vi "LIA_FPGA.vi"() -> ()   [LabVIEW 2009]
uses:
  <vilib>/LabVIEW Targets/FPGA/cRIO/shared/nicrio_ModuleControls/nicrio_cRIO-9233_DataRatesRing.ctl
  <vilib>/rvi/LocalResourceManager/LocalResourceManager.xnode
  <vilib>/rvi/eio/common/nirviEmuReportErrorAndStop.vi
  <vilib>/rvi/DataTransferAndStorage/Container/Common/niFpgaContainerSetEmuInfo.vi
  <vilib>/rvi/DataTransferAndStorage/Container/Common/niFpgaContainerState.ctl
  <vilib>/rvi/DataTransferAndStorage/Container/Common/niFpgaDataTypeControl.ctl
  <vilib>/rvi/DataTransferAndStorage/Container/Common/niFpgaContainerImplementationControl.ctl
  <vilib>/rvi/DataTransferAndStorage/Container/Common/niFpgaContainerArbitrationOptionsControl.ctl
  <vilib>/rvi/DataTransferAndStorage/Container/Common/niFpgaTransferTypeControl.ctl
  <vilib>/rvi/DataTransferAndStorage/Container/Common/niFpgaContainerInitializationParameters.ctl
  <vilib>/rvi/DataTransferAndStorage/Container/Common/niFpgaContainerMetaDataKey.ctl
  <vilib>/eio/EIOPropertyNode/EIOPropertyNode.xnode
  <vilib>/rvi/eio/nirviEIOPropertyImplementation/nirviEIOPropertyImplementation.xnode
  <vilib>/rvi/eio/common/nirviEmuTemplatePropertyGet_noerrors.vi
  <vilib>/rvi/eio/common/nirviEmuTemplatePropertySet_noerrors.vi
  <vilib>/eio/EIONode/EIONode.xnode
  <vilib>/rvi/eio/nirviEIOImplementation/nirviEIOImplementation.xnode
  <vilib>/rvi/eio/common/nirviEmuTemplateMethod_noerrors.vi
  <vilib>/rvi/eio/common/nirviEmuClasses.ctl
  <vilib>/Platform/TimedLoop/XDataNode/XDataNode.xnode
  <vilib>/Platform/TimedLoop/XDataNode/loadlvalarms.vi
  <vilib>/Platform/TimedLoop/XDataNode/timing_clust.ctl
  <vilib>/Platform/TimedLoop/XDataNode/nitl_modes.ctl
  <vilib>/Platform/TimedLoop/XDataNode/wakeup.ctl
  <vilib>/rvi/DataTransferAndStorage/Container/XNode/niFpgaContainer.xnode
  <vilib>/rvi/FIFO/Fifo_Resource/nirvififoUniquifyingName.vi
  <vilib>/rvi/FXPMathLib/FxpSinAndCos/XNode/nifxpmath_SinAndCos.xnode
  <vilib>/rvi/FXPMathLib/FxpSinAndCos/subVIs/nifxpmath_SinAndCos_SimConfig.ctl
  <vilib>/rvi/FXPMathLib/FxpSinAndCos/simVIs/DllFxpSinAndCosTemp_sub.vi
  <vilib>/rvi/interface/RandomDataEmulation/niFpgaRandomDataHandleErrors.vi
  <vilib>/rvi/interface/RandomDataEmulation/nirviRandomDataFPGAFIFO.vi
  <vilib>/rvi/DataTransferAndStorage/Container/Common/niFpgaContainerMethod.ctl
  <vilib>/Platform/TimedLoop/XDataNode/XDNodeRunTimeDep.lvlib
panel:
  in  "dec":i32
  out "channelQ":i64
  out "channelI":i64
  in  "reset":bool
  in  "Data Rate":T1=2 items=["50.000 kS/s (NI 9233)"=2, "33.333 kS/s (NI 9233)"=3, "25.000 kS/s (NI 9233)"=34, "16.667 kS/s (NI 9233)"=35, "12.500 kS/s (NI 9233)"=36, "10.000 kS/s (NI 9233)"=37, "  8.333 kS/s (NI 9233)"=38, "  7.143 kS/s (NI 9233)"=39, "  6.250 kS/s (NI 9233)"=40, "  5.556 kS/s (NI 9233)"=41, "  5.000 kS/s (NI 9233)"=42, "  4.545 kS/s (NI 9233)"=43, "  4.167 kS/s (NI 9233)"=44, "  3.846 kS/s (NI 9233)"=45, "  3.571 kS/s (NI 9233)"=46, "  3.333 kS/s (NI 9233)"=47, "  3.125 kS/s (NI 9233)"=48, "  2.941 kS/s (NI 9233)"=49, "  2.778 kS/s (NI 9233)"=50, "  2.632 kS/s (NI 9233)"=51, "  2.500 kS/s (NI 9233)"=52, "  2.381 kS/s (NI 9233)"=53, "  2.273 kS/s (NI 9233)"=54, "  2.174 kS/s (NI 9233)"=55, "  2.083 kS/s (NI 9233)"=56, "  2.000 kS/s (NI 9233)"=57]
  out "f_2":fxp<+/-,32,0> format="%.32g"
  out "f":fxp<+/-,32,0> format="%.32g"
  out "Offset":i32
  out "LSB Weight":u32
  in  "channel":i16
  in  "test":bool
  out "error":bool
  in  "dec2":i16
  in  "K":fxp<+,16,0>
  in  "nominal freq":fxp<+,16,0>
  in  "dec1":i16
  in  "stages":i8=1
  in  "stop":bool
  in  "decimation":i16=1024
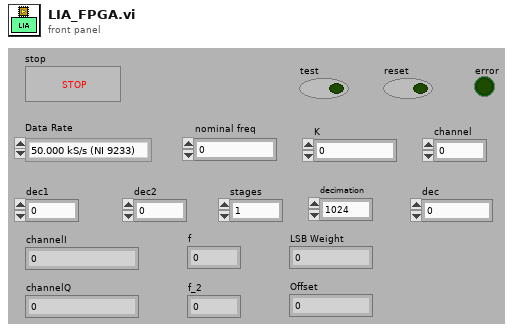
[diagram p1: front panel]
types:
  T1 = typedef "nicrio_cRIO-9233_DataRatesRing.ctl" = u8
  T2 = typedef "nirviEmuClasses.ctl" = enum16{"IO Read", "IO Write", "Method", "Property Read", "Property Write"}
  T3 = typedef "XDNodeRunTimeDep.lvlib/timing_clust.ctl" = cluster{"Expected End [f-1]":u64, "Actual End [f-1]":u64, "Finished Late? [f-1]":bool, "Expected End [i-1]":u64, "Actual End [i-1]":u64, "Finished Late? [i-1]":bool, "Expected Start [i]":u64, "Actual Start [i]":u64, "Expected Start [f]":u64, "Actual Start [f]":u64, "Source Name":string, "Structure Name":string, "Period":i64, "Deadline":i64, "Offset":i64, "Start":i64, "Priority":i32, "Timeout":i32, "Mode":T4, "Wakeup Reason":T5, "Error":errorcluster, "Source Type":string, "Secondary Source Type":string, "Global End Time":u64, "Global Start Time":u64, "Frame Duration":u64, "Iteration Duration":u64, "Assigned CPU":i32, "I/O Scan Engine Mode":u32}
  T4 = typedef "XDNodeRunTimeDep.lvlib/nitl_modes.ctl" = enum32{"No Change", "Process missed periods, maintain original phase", "Discard missed periods, maintain original phase", "Process missed periods, ignore original phase", "Discard missed periods, ignore original phase"}
  T5 = typedef "XDNodeRunTimeDep.lvlib/wakeup.ctl" = enum32{"Normal", "Aborted", "Asynchronous wakeup", "Timing source error", "Timed loop error", "Timeout"}
  T6 = typedef "niFpgaContainerMethod.ctl" = enum16{"Write", "Read", "Clear", "Get Number of Elements to Write", "Get Number of Elements to Read", "Enable", "Disable", "Flush and Disable", "Get Stream State"}
  T7 = typedef "niFpgaTransferTypeControl.ctl" = enum16{"Target-Scoped", "Host to Target - DMA", "Target to Host - DMA", "Peer to Peer Reader", "Peer to Peer Writer", "Bidirectional"}
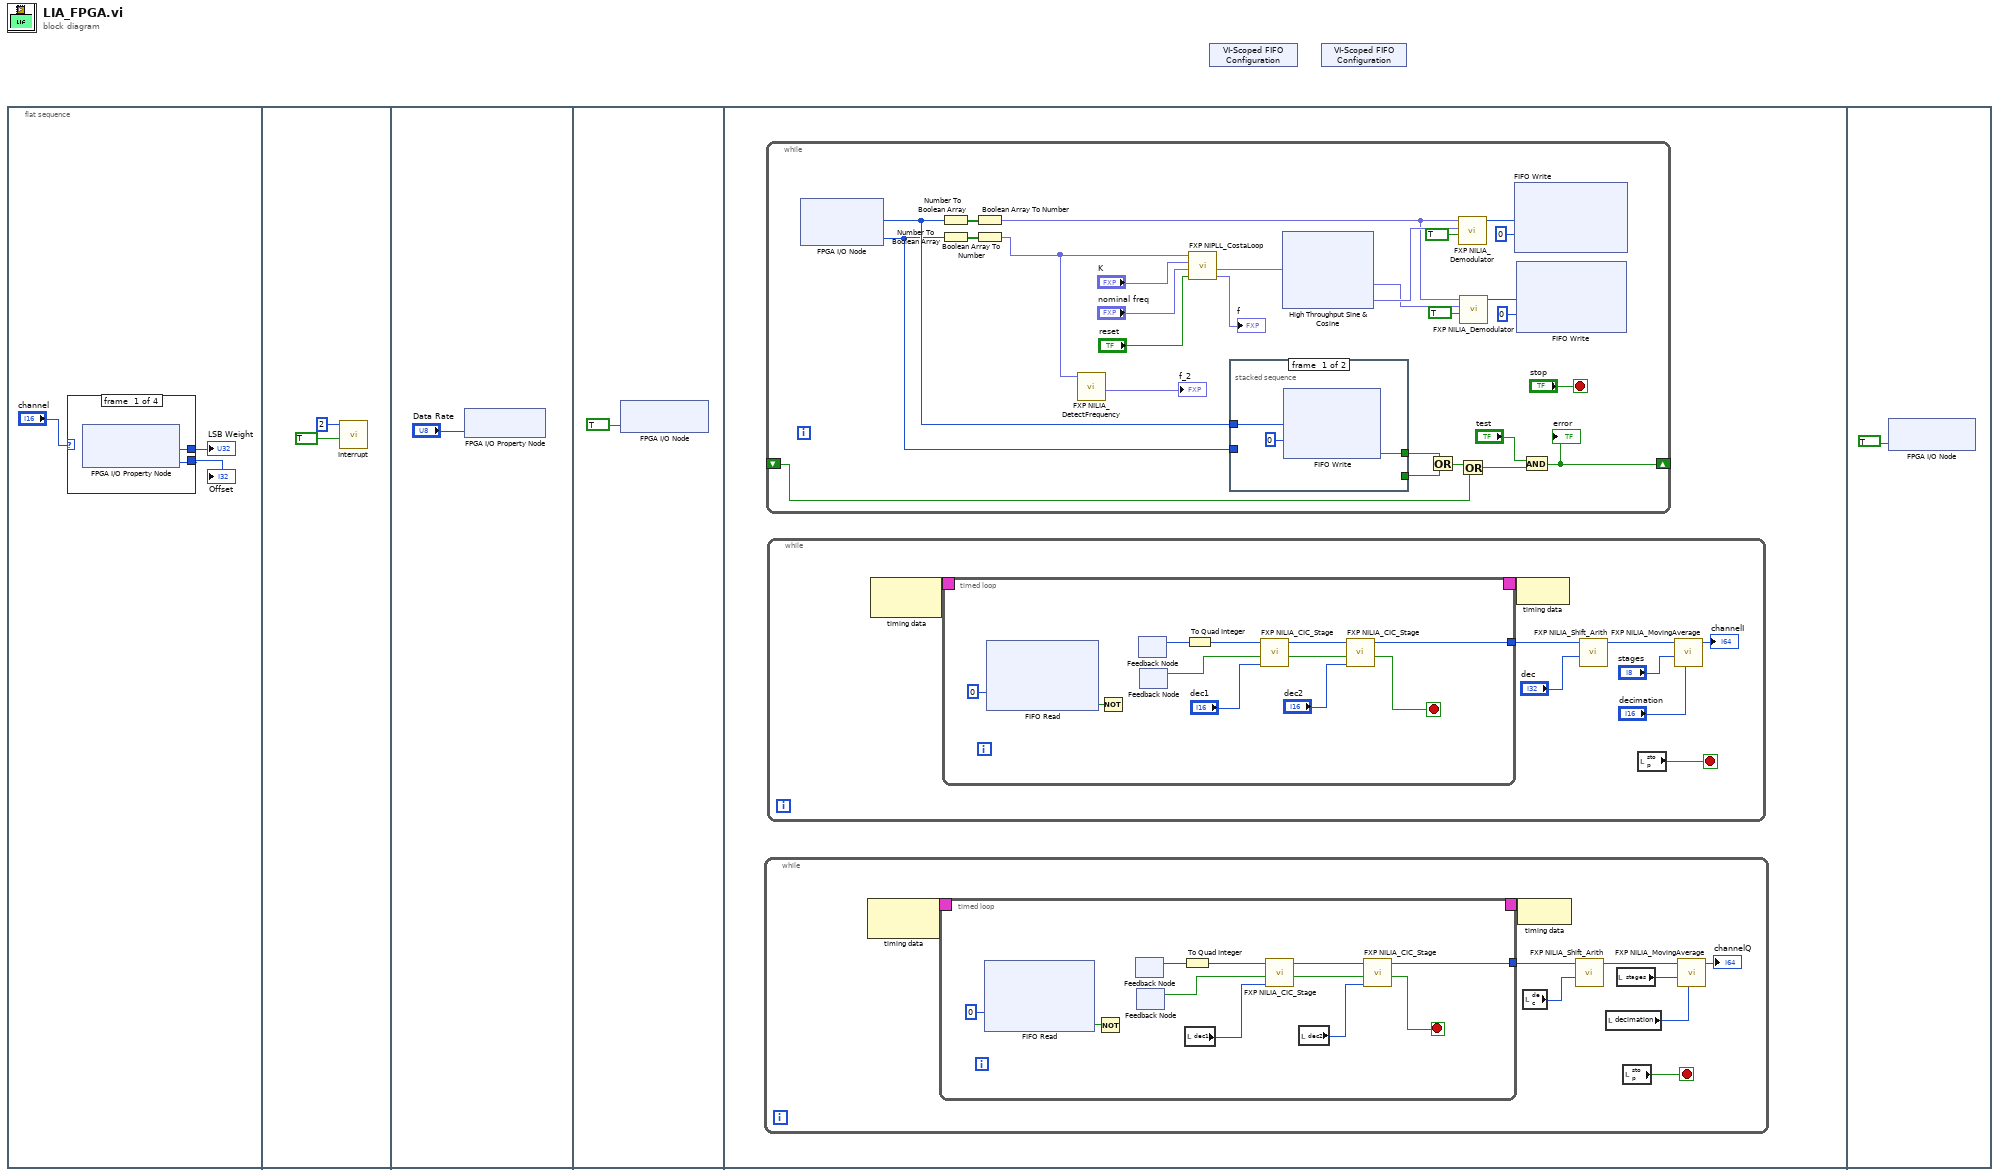
[diagram p0: block diagram]
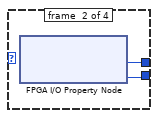
[diagram p2: hidden frame]
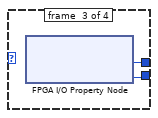
[diagram p3: hidden frame]
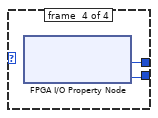
[diagram p4: hidden frame]
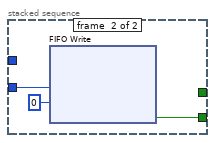
[diagram p5: hidden frame]
diagram:
  n1 = flat-sequence {
    frame #0 {
      n2 = case shown="0, Default" "channel" {
        tunnel: [w5 w38 w71 w104] -> w2
        tunnel: [w4 w37 w70 w103] -> w1
        frame #0 {
          n3 = xnode "FPGA I/O Property Node"() -> ("LSB Weight"=w5:u32, "Offset"=w4:i32)  [unwired: 1 in, 1 out]
        }
        frame #1 {
          n4 = xnode "FPGA I/O Property Node"() -> ("LSB Weight"=w38:u32, "Offset"=w37:i32)  [unwired: 1 in, 1 out]
        }
        frame #2 {
          n5 = xnode "FPGA I/O Property Node"() -> ("LSB Weight"=w71:u32, "Offset"=w70:i32)  [unwired: 1 in, 1 out]
        }
        frame #3 {
          n6 = xnode "FPGA I/O Property Node"() -> ("LSB Weight"=w104:u32, "Offset"=w103:i32)  [unwired: 1 in, 1 out]
        }
      }
      "LSB Weight" <- w2
      "Offset" <- w1
    }
    frame #1 {
      n7 = call "Interrupt"("Wait Until Cleared"=TRUE, "IRQ Number"=u8 2) -> ()  [unwired: 1 out]
    }
    frame #2 {
      n8 = xnode "FPGA I/O Property Node"("Data Rate"="Data Rate") -> ()  [unwired: 1 in, 1 out]
    }
    frame #3 {
      n9 = xnode "FPGA I/O Node"("Mod1/Start"=TRUE) -> ()  [unwired: 1 in, 1 out]
    }
    frame #4 {
      n10 = while {
        stop <- w163 stop-if-true
        n11 = node-c288() -> (w165:T3)  [unwired: 1 in]
        n12 = timed-loop {
          timing: w165 -> [_]
          timing-out: [_] -> w164
          tunnel: [w167] -> w162
          stop <- w166 stop-if-true
          n13 = xnode ("FIFO Read")("Timeout"=0) -> ("Element"=w176:i32, "Timed Out?"=w175:bool)  [unwired: 1 in, 1 out]
          n14 = Not(x=w175) -> (.not. x?=w174:bool)
          n15 = feedback #1() -> (w178:i32)  [unwired: 1 in]
          n16 = feedback #2() -> (w172:bool)  [unwired: 1 in]
          n17 = To Quad Integer(1:w178) -> (0:w173:i64)
          n18 = local read "dec1"() -> (w171:i16)
          n19 = call "FXP NILIA_CIC_Stage.vi"("decimate factor"=w171, "New Data"=w172, "input"=w173) -> ("Data Ready"=w169:bool, "output"=w170:i64)  [unwired: 7 in]
          n20 = local read "dec2"() -> (w168:i16)
          n21 = call "FXP NILIA_CIC_Stage.vi"("decimate factor"=w168, "New Data"=w169, "input"=w170) -> ("Data Ready"=w166:bool, "output"=w167:i64)  [unwired: 7 in]
        }
        n22 = node-c288(w164) -> ()
        n23 = local read "dec"() -> (w161:i32)
        n24 = call "FXP NILIA_Shift_Arith.vi"("dec"=w161, "x"=w162) -> ("y"=w160:i64)  [unwired: 9 in]
        n25 = local read "decimation"() -> (w158:i16)
        n26 = local read "stages"() -> (w159:i8)
        n27 = local read "stop"() -> (w163:bool)
        n28 = call "FXP NILIA_MovingAverage.vi"("decimate"=w158, "stages"=w159, "input"=w160) -> ("output"=→"channelQ":i64)  [unwired: 8 in]
      }
      n29 = while {
        shift-right: [w251] -> _
        shift-left: _ -> [w231]
        stop <- "stop" stop-if-true
        n30 = xnode "FPGA I/O Node"() -> ("Mod1/AI0"=w242:i32, "Mod1/AI1"=w241:i32)  [unwired: 2 in, 2 out]
        n31 = Number To Boolean Array(number=w242) -> (Boolean array=w244:bool[])
        n32 = Number To Boolean Array(number=w241) -> (Boolean array=w243:bool[])
        n33 = Boolean Array To Number(Boolean array=w244) -> (number=w235:fxp<+/-,24,1>)
        n34 = Boolean Array To Number(Boolean array=w243) -> (number=w240:fxp<+/-,24,1>)
        n35 = call "FXP NILIA_DetectFrequency.vi"("x"=w240) -> ("f_2"=→"f_2":fxp<+/-,32,0>)  [unwired: 9 in, 1 out]
        n36 = call "FXP NIPLL_CostaLoop.vi"("reset?"="reset", "norminal freq [U16.0]"="nominal freq", "alpha [U16.0]"="K", "x[I24.1]"=w240) -> ("f"=→"f":fxp<+/-,32,0>, "z [I32.1]"=w248:fxp<+/-,32,1>)  [unwired: 4 in, 2 out]
        n37 = stacked-sequence {
          tunnel: w242 -> [w424 _]
          tunnel: w241 -> [_ w452]
          tunnel: [w423 _] -> w256
          tunnel: [_ w451] -> w255
          frame #0 {
            n38 = xnode ("FIFO Write")("Element"=w424, "Timeout"=0) -> ("Timed Out?"=w423:bool)  [unwired: 1 in, 1 out]
          }
          frame #1 {
            n39 = xnode ("FIFO Write")("Element"=w452, "Timeout"=0) -> ("Timed Out?"=w451:bool)  [unwired: 1 in, 1 out]
          }
        }
        n40 = xnode "High Throughput Sine & Cosine"("x (pi)"=w248) -> ("sin(x)"=w234:fxp<+/-,24,2>, "cos(x)"=w238:fxp<+/-,24,2>)
        n41 = Or(x=w256, y=w255) -> (x .or. y?=w254:bool)
        n42 = call "FXP NILIA_Demodulator.vi"("New Data"=TRUE, "ref"=w238, "signal"=w235) -> ("x*y"=w236:i32)  [unwired: 7 in, 1 out]
        n43 = call "FXP NILIA_Demodulator.vi"("New Data"=TRUE, "ref"=w234, "signal"=w235) -> ("x*y"=w232:i32)  [unwired: 7 in, 1 out]
        n44 = Or(x=w254, y=w231) -> (x .or. y?=w253:bool)
        n45 = xnode ("FIFO Write")("Element"=w236, "Timeout"=0) -> ()  [unwired: 1 in, 2 out]
        n46 = xnode ("FIFO Write")("Element"=w232, "Timeout"=0) -> ()  [unwired: 1 in, 2 out]
        n47 = And(x="test", y=w253) -> (x .and. y?=w251:bool)
        "error" <- w251
      }
      n48 = while {
        stop <- w485 stop-if-true
        n49 = node-c288() -> (w487:T3)  [unwired: 1 in]
        n50 = timed-loop {
          timing: w487 -> [_]
          timing-out: [_] -> w486
          tunnel: [w489] -> w484
          stop <- w488 stop-if-true
          n51 = xnode ("FIFO Read")("Timeout"=0) -> ("Element"=w498:i32, "Timed Out?"=w497:bool)  [unwired: 1 in, 1 out]
          n52 = Not(x=w497) -> (.not. x?=w496:bool)
          n53 = feedback #3() -> (w500:i32)  [unwired: 1 in]
          n54 = feedback #4() -> (w494:bool)  [unwired: 1 in]
          n55 = To Quad Integer(1:w500) -> (0:w495:i64)
          n56 = call "FXP NILIA_CIC_Stage.vi"("decimate factor"="dec1", "New Data"=w494, "input"=w495) -> ("Data Ready"=w491:bool, "output"=w492:i64)  [unwired: 7 in]
          n57 = call "FXP NILIA_CIC_Stage.vi"("decimate factor"="dec2", "New Data"=w491, "input"=w492) -> ("Data Ready"=w488:bool, "output"=w489:i64)  [unwired: 7 in]
        }
        n58 = node-c288(w486) -> ()
        n59 = call "FXP NILIA_Shift_Arith.vi"("dec"="dec", "x"=w484) -> ("y"=w482:i64)  [unwired: 9 in]
        n60 = local read "stop"() -> (w485:bool)
        n61 = call "FXP NILIA_MovingAverage.vi"("decimate"="decimation", "stages"="stages", "input"=w482) -> ("output"=→"channelI":i64)  [unwired: 8 in]
      }
    }
    frame #5 {
      n62 = xnode "FPGA I/O Node"("Mod1/Stop"=TRUE) -> ()  [unwired: 1 in, 1 out]
    }
  }
  n63 = xnode "VI-Scoped FIFO Configuration"() -> ()  [unwired: 1 out]
  n64 = xnode "VI-Scoped FIFO Configuration"() -> ()  [unwired: 1 out]
